vi "tm_setoutputtrigger.vi"(8 "error in (no error)":errorcluster, 9 "Index":i32, 10 "Parameters":T1={"Mode"=1, "Polarity"=1, "Period"=0.0, "Delay"=0.0} {"Polarity" items=["Negative"=1, "Positive"=2]; "Mode" items=["Low"=1, "Global Exposure"=2, "Programmable"=3, "Trigger Ready"=4, "High"=5]}, 11 "Handle in":u32) -> (0 "error out":errorcluster, 3 "Handle out":u32)   [LabVIEW 2023]
uses:
  tmcamcon.dll
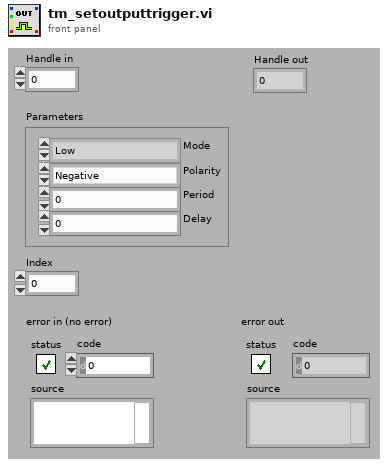
[diagram p1: front panel]
types:
  T1 = cluster{"Mode":u32, "Polarity":u32, "Period":dbl, "Delay":dbl}
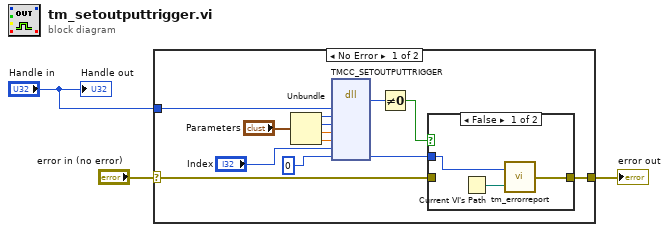
[diagram p0: block diagram]
diagram:
  n1 = case shown="No Error" "error in (no error)" {
    selector: "error in (no error)" -> [w7 w21]
    tunnel: [w4 w21] -> w2
    tunnel: "Handle in" -> [w12 _]
    frame No Error {
      n2 = Unbundle("Parameters") -> ("Mode"=w11:u32, "Polarity"=w10:u32, "Period"=w9:dbl, "Delay"=w8:dbl)
      n3 = dll-call lib="tmcamcon.dll" fn="TMCC_SETOUTPUTTRIGGER"("HDCAM"=w12, "mode"=w11, "polarity"=w10, "period"=w9, "delay"=w8, "index"="Index", "Erval"=0) -> ("return type"=w16:u32, "Erval"=w6:i32)  [unwired: 9 in, 2 out]
      n4 = Not Equal To 0?(x=w16) -> (x != 0?=w5:bool)
      n5 = case shown="False" w5 {
        tunnel: w7 -> [_ w20]
        tunnel: [w18 w20] -> w4
        tunnel: w6 -> [w17 _]
        frame False {
          n6 = Current VI's Path() -> (path=w19:path)
          n7 = call "tm_errorreport.vi"("Source"=w19, "Error"=w17) -> ("error out"=w18:errorcluster)
        }
        frame True {
        }
      }
    }
    frame Error {
    }
  }
  "error out" <- w2
  "Handle out" <- "Handle in"
